vi "Get Updated.vi"(8 "error in (no error)":errorcluster, 11 "ViaApp in":refnum<class "ViaApp.lvclass">) -> (0 "error out":errorcluster, 2 "Last Update":timestamp, 3 "ViaApp out":refnum<class "ViaApp.lvclass">)   [LabVIEW 2020, in "PicoG-App.lvlib" / "ViaApp.lvclass"]
uses:
  ViaApp.lvclass
  ViaApp.lvclass/ViaApp.ctl
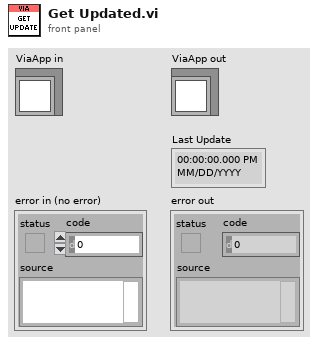
[diagram p1: front panel]
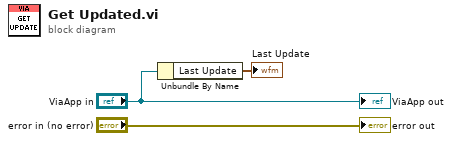
[diagram p0: block diagram]
diagram:
  n1 = Unbundle By Name("ViaApp in") -> ("Last Update"=→"Last Update":timestamp)
  "error out" <- "error in (no error)"
  "ViaApp out" <- "ViaApp in"
